vi "SlotNum Write.vi"(4 "error in (no error)":errorcluster, 5 "Value":i32, 6 "Container State":T2, 7 "Display State In":T1) -> (0 "error out":errorcluster, 3 "Display State Out":T1)   [LabVIEW 2015, in "Digital I-O.xctl"]
uses:
  Digital I-O.xctl
  <vilib>/_xctls/Container State.ctl
  State.ctl
  <vilib>/_xctls/XControlSupport.lvlib
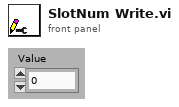
[diagram p1: front panel]
types:
  T1 = typedef "Digital I-O.xctl/State.ctl" = cluster{"Hide unused":bool, "Is dirty?":bool, "SlotNum":i32, "Output List":string[], "Input List":string[]}
  T2 = typedef "XControlSupport.lvlib/Container State.ctl" = cluster{"Indicator?":bool, "Run Mode?":bool, " Refnum":refnum<vi>}
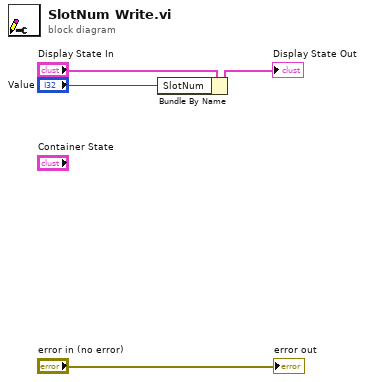
[diagram p0: block diagram]
diagram:
  n1 = Bundle By Name(cluster="Display State In", "SlotNum"="Value") -> (→"Display State Out":T1)
  "error out" <- "error in (no error)"
